vi "mess返回值解析.vi"(11 "ValidateBarcode":string="True,10458935,C.0C.01B,Firebird2药物支架系统（无标签）G2513,G2513,5") -> (3 "元素":string)   [LabVIEW 2017]
panel:
  out "数组":string[](array[string])
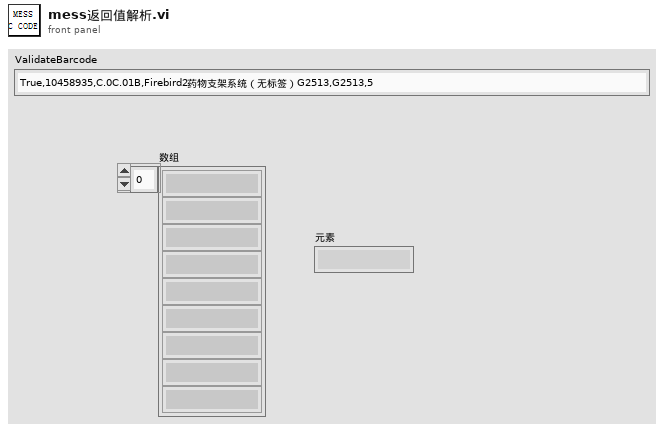
[diagram p1: front panel]
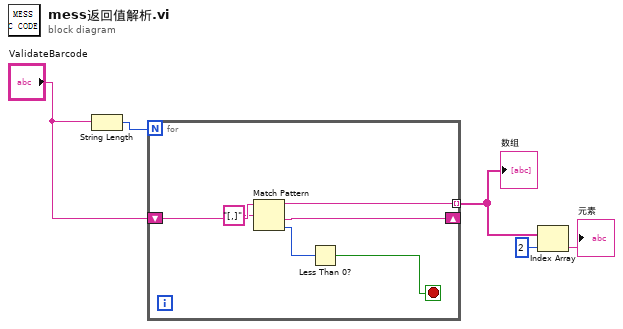
[diagram p0: block diagram]
diagram:
  n1 = String Length(string="ValidateBarcode") -> (length=w4:i32)
  n2 = for {
    N: w4 -> [_]
    tunnel: [w7] -> w3 mode=indexing
    shift-right: [w6] -> _
    shift-left: "ValidateBarcode" -> [w11]
    stop <- w8 stop-if-true
    n3 = Match Pattern(string=w11, regular expression="[,]" ("正则表达式")) -> (before substring=w7:string, after substring=w6:string, offset past match=w9:i32)  [unwired: 1 in, 1 out]
    n4 = Less Than 0?(x=w9) -> (x < 0?=w8:bool)
  }
  "数组" <- w3
  n5 = Index Array(array=w3, index=2 ("索引")) -> (element=→"元素":string)
